vi "ini_save_cplx_double_vector.vi"(7 "section":string, 8 "error in":errorcluster, 9 "values":cdb[](array[numeric]), 10 "key":string, 11 "refnum in":T1) -> (0 "error out":errorcluster, 2 "found?":bool, 3 "refnum out":T1)   [LabVIEW 2013]
uses:
  <vilib>/Utility/config.llb/Config Data RefNum.ctl
  <vilib>/Utility/config.llb/Write Key (String).vi
  <vilib>/Utility/config.llb/NI_LVConfig.lvlib
panel:
  out "trimmed string":string
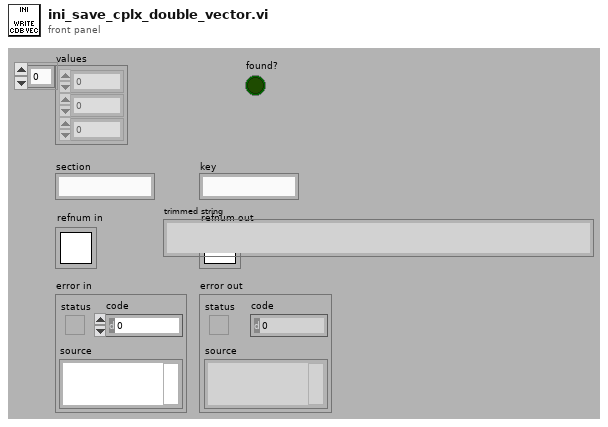
[diagram p1: front panel]
types:
  T1 = typedef "NI_LVConfig.lvlib/Config Data RefNum.ctl" = refnum<k1>
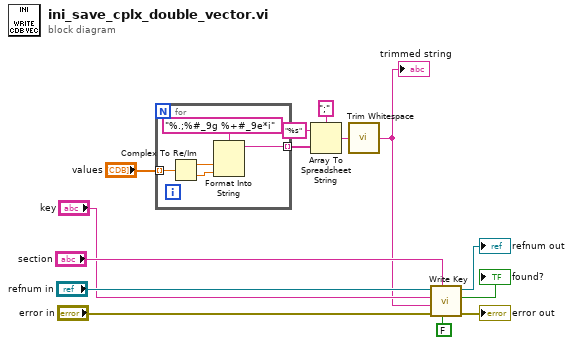
[diagram p0: block diagram]
diagram:
  n1 = for {
    tunnel: "values" -> [w19] mode=indexing
    tunnel: [w15] -> w5 mode=indexing
    n2 = Complex To Re/Im(x + iy=w19) -> (x=w18:dbl, y=w17:dbl)
    n3 = Format Into String(format string="%.;%#_9g %+#_9e*i", w18, w17) -> (resulting string=w15:string)  [unwired: 2 in, 1 out]
  }
  n4 = Array To Spreadsheet String(delimiter (Tab)=";", array=w5, 3:"%s" ("format string")) -> (spreadsheet string=w2:string)
  n5 = call <vilib>:"Trim Whitespace.vi"("string"=w2) -> ("trimmed string"=w1:string)  [unwired: 1 in]
  "trimmed string" <- w1
  n6 = call-poly <vilib>:"Write Key.vi"("write raw string? (F)"=FALSE, "section"="section", "error in (no error)"="error in", "value"=w1, "key"="key", "refnum"="refnum in") -> ("error out"=→"error out":errorcluster, "found?"=→"found?":bool, "refnum out"=→"refnum out":T1)  [unwired: 3 in]
